vi "Command Editor Dialog.vi"(7 "Name (\"\" to Use Uuid)":string="Event CSM Tiny", 8 "Error In":errorcluster caption="Error in (no error)", 11 "CSM States":string="UI: Front Panel State >> Open -@ abc") -> (0 "Error Out":errorcluster, 3 "Command Out":string)   [LabVIEW 2017]
uses:
  _Support/Single-Line Type.ctl
  _Support/CSM Part Property.ctl
  _Support/Single-Line Selection Type.ctl
  <vilib>/Utility/miscctls.llb/LVRowAndColumnUnsignedTypeDef.ctl
  _Shared/Trim Single-line Text.vi
  AdvanceAPI/CSM - Break Down Multiple States String.vi
  AdvanceAPI/CSM - Compact Multiple States.vi
  AdvanceAPI/CSM - Keywords.vi
  _Polymophic/CSM - Filter Duplicated Lines.vi
  Communicable State Machine.lvlib
  _Shared/CSM Shared.lvlib
panel:
  out "MsgType":string
  out "Selction":string
  out "SelType":string
  out "Ref-String":string
  in  "clear arguments":bool
  in  "->|":bool
  in  "->":bool
  in  "-@":bool
  in  "Candidates":i32(listbox)
  # "Flood of Events:\n\nPanel/Pane Size Event\nSlide/Knob... User Event by dragging\nNumeric Control Value Change Event by Arraw Button"
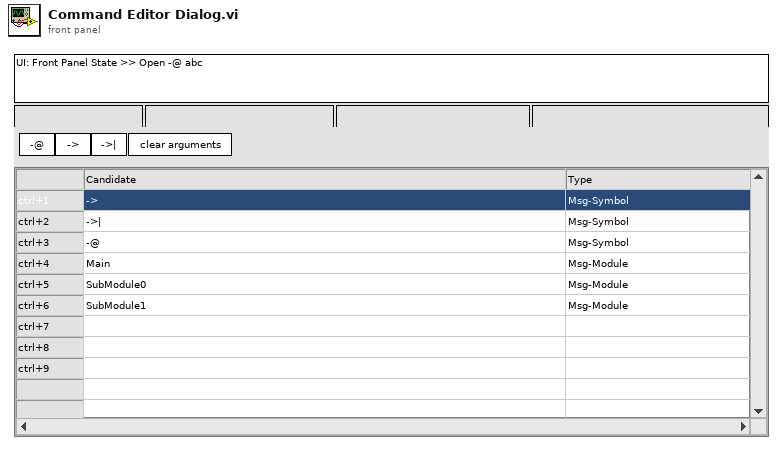
[diagram p1: front panel]
types:
  T1 = enum32{"Invalid", "Standard", "Closed", "Hidden", "Minimized", "Maximized"}
  T2 = enum32{"invalid app kind", "Development System", "Run Time System", "Student Edition", "Embedded LabVIEW", "Evaluation", "Custom"}
  T3 = typedef "LVRowAndColumnUnsignedTypeDef.ctl" = cluster{"Row":u32, "Column":u32}
  T4 = typedef "Communicable State Machine.lvlib/_CSM_Response Source Message.ctl" = cluster{"‘State":string, "’Arguments":string, "’Error":errorcluster}
  T5 = cluster{"Current VI Reference":refnum<vi>, "Close Panel on Exit?":bool}
  T6 = typedef "CSM Part Property.ctl" = cluster{"Section Start":u32, "Section End":u32, "Start":u32, "End":u32, "Section":string, "Core":string, "Sel Type":T7, "Ref-String":string}
  T7 = typedef "Single-Line Selection Type.ctl" = enum16{"<unknown>", "Reg-SourceSignal", "Reg-@Seperator", "Reg-ArgSymbol", "Reg-TargetAPI", "Reg-Module", "Reg-Symbol", "Reg-Oper", "Msg-State", "Msg-Arg", "Msg-ArgSymbol", "Msg-Symbol", "Msg-Module", "Broadcast-Signal", "Broadcast-ArgSymbol", "Broadcast-Arg", "Broadcast-Symbol", "Broadcast-Oper", "Comment-Symbol", "Comment-Content"}
  T8 = typedef "Single-Line Type.ctl" = enum16{"Message", "Broadcast", "Registration"}
  T9 = cluster{"Core":cluster{"Current VI Reference":refnum<vi>, "Close Panel on Exit?":bool}, "CSM States":string, "Selection":T6[], "Msg Type":T8}
  T10 = typedef "LVSelectionTypeDef.ctl" = cluster{"Selection Start":u32, "Selection End":u32}
  T11 = typedef "eventvkey.ctl" = enum16{"ASCII", "Enter", "Return", "Shift", "Ctrl", "Alt", "Cmd", "Opt", "Caps", "NumLock", "Clear", "Break", "Up", "Down", "Left", "Right", "Insert", "Delete", "Home", "End", "PageUp", "PageDown", "Escape", "Help", "Pause", "ScrollLock", "F1", "F2", "F3", "F4", "F5", "F6", "F7", "F8", "F9", "F10", "F11", "F12", "F13", "F14", "F15", "F16", "F17", "F18", "F19", "F20", "F21", "F22", "F23", "F24", "Play", "VolumeUp", "VolumeDown", "Mute", "Two Byte Char"}
  T12 = cluster{"Shift":bool, "Ctrl":bool, "Alt":bool, "Cmd":bool, "Opt":bool}
  T13 = typedef "LVPoint32TypeDef.ctl" = cluster{"Horizontal":i32, "Vertical":i32}
  T14 = typedef "LVRowAndColumnTypeDef.ctl" = cluster{"Row":i32, "Column":i32}
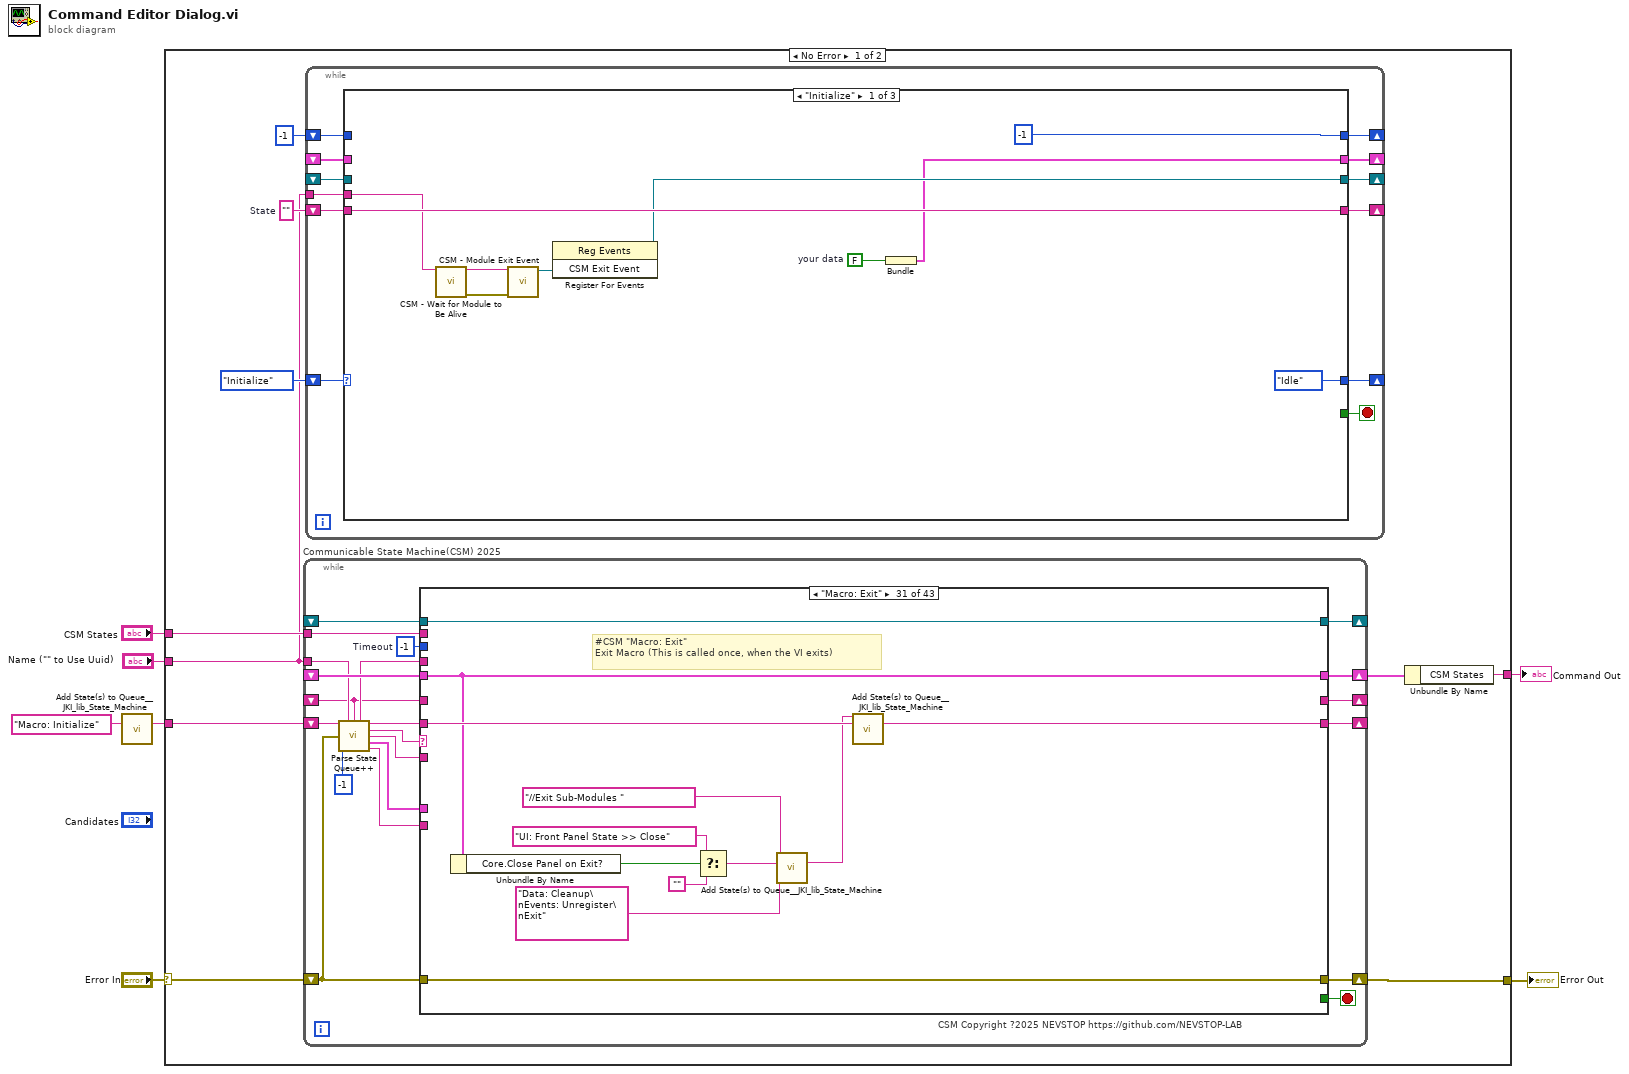
[diagram p0: block diagram]
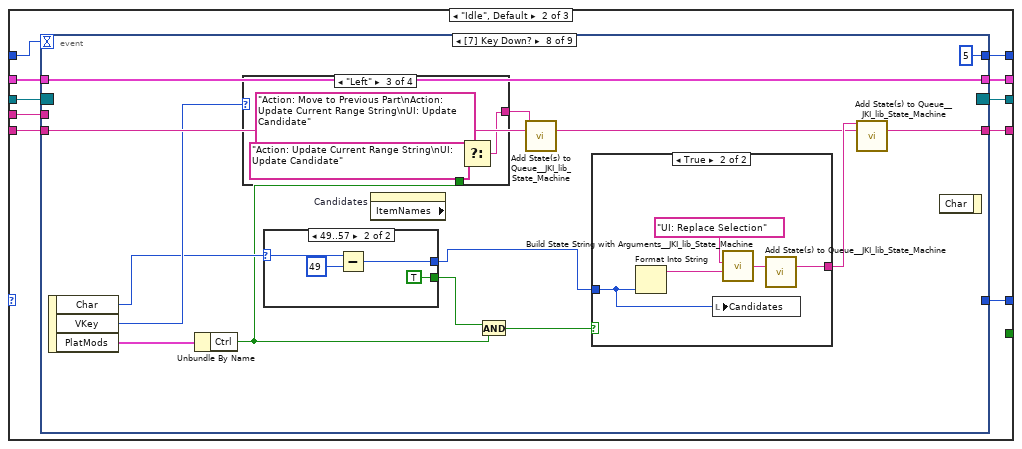
[diagram p2: hidden frame]
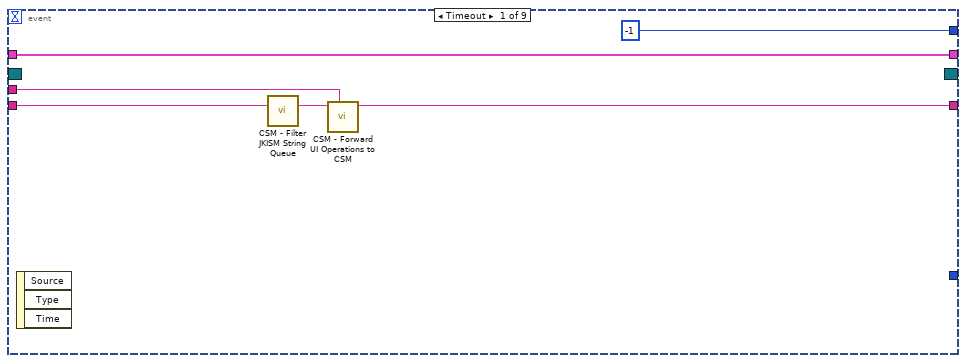
[diagram p3: hidden frame]
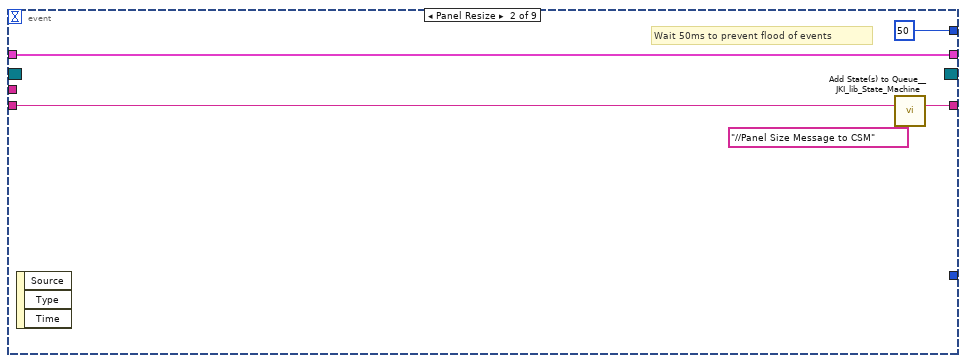
[diagram p4: hidden frame]
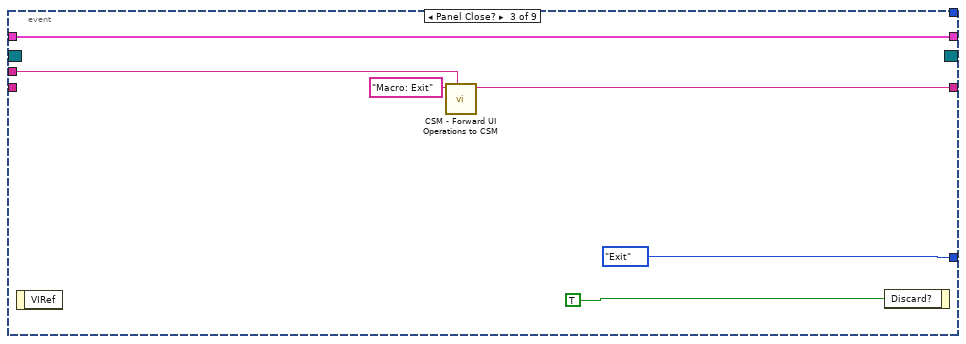
[diagram p5: hidden frame]
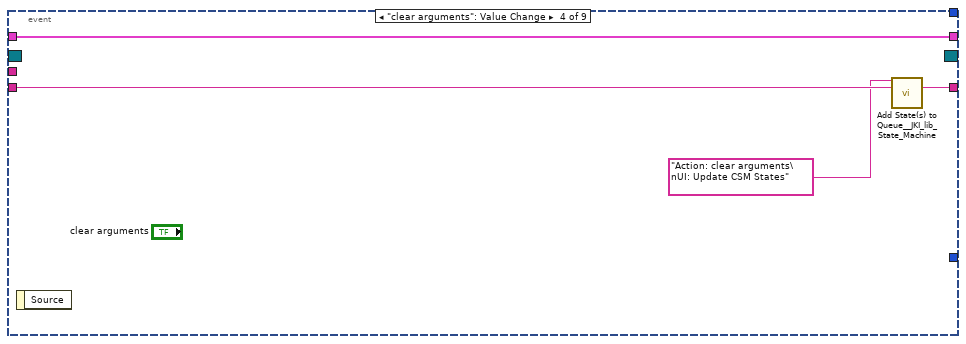
[diagram p6: hidden frame]
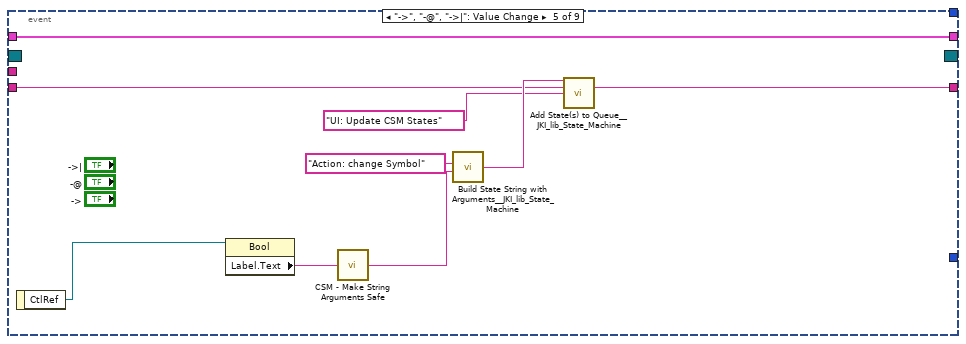
[diagram p7: hidden frame]
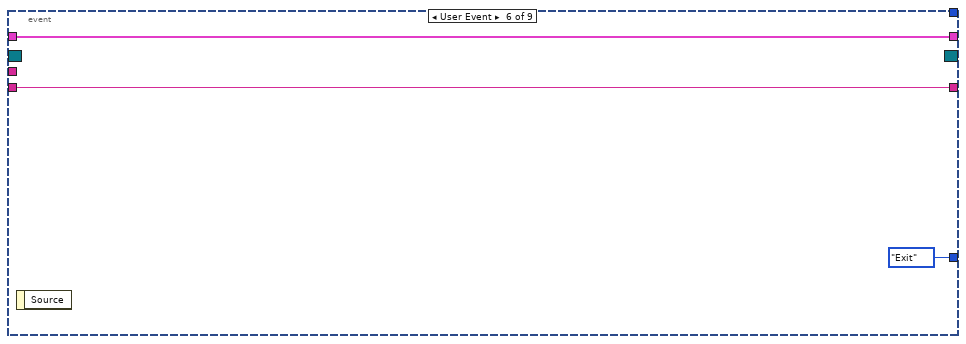
[diagram p8: hidden frame]
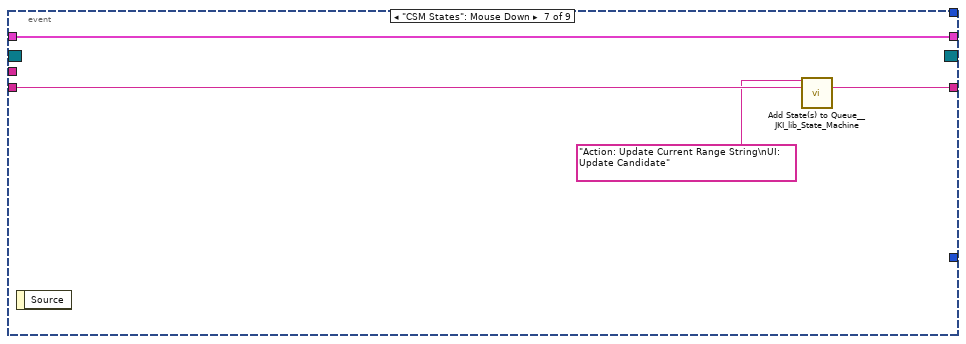
[diagram p9: hidden frame]
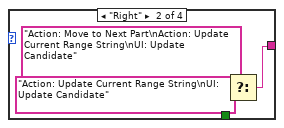
[diagram p11: hidden frame]
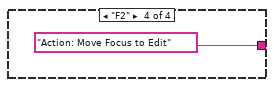
[diagram p12: hidden frame]
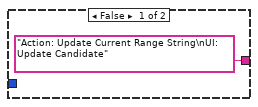
[diagram p13: hidden frame]
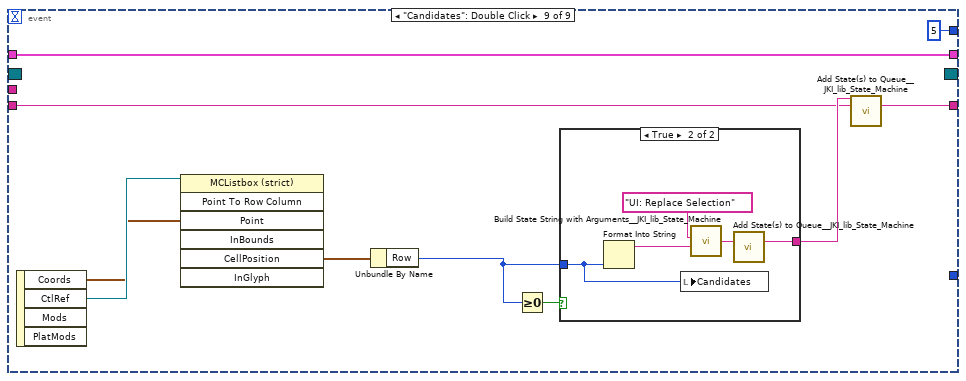
[diagram p15: hidden frame]
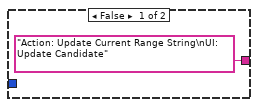
[diagram p16: hidden frame]
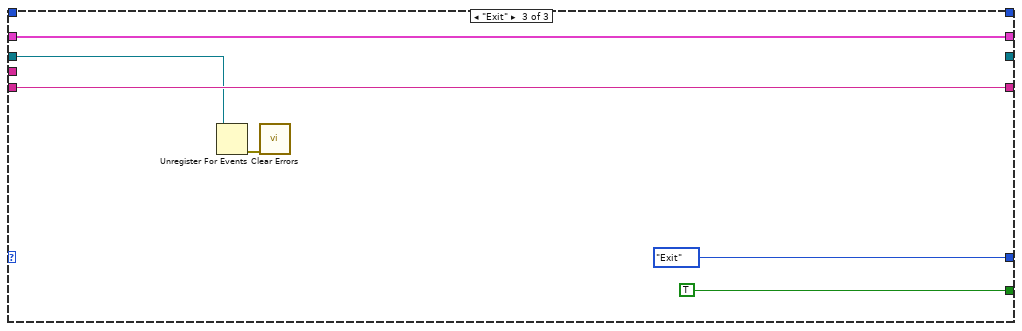
[diagram p17: hidden frame]
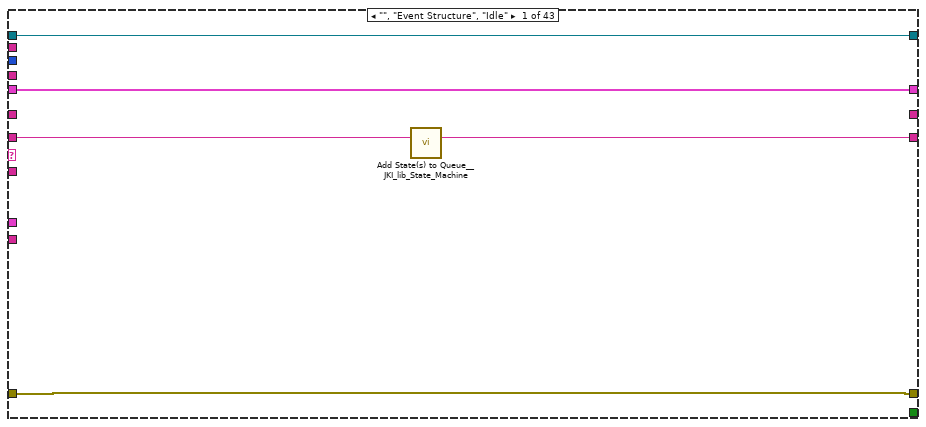
[diagram p18: hidden frame]
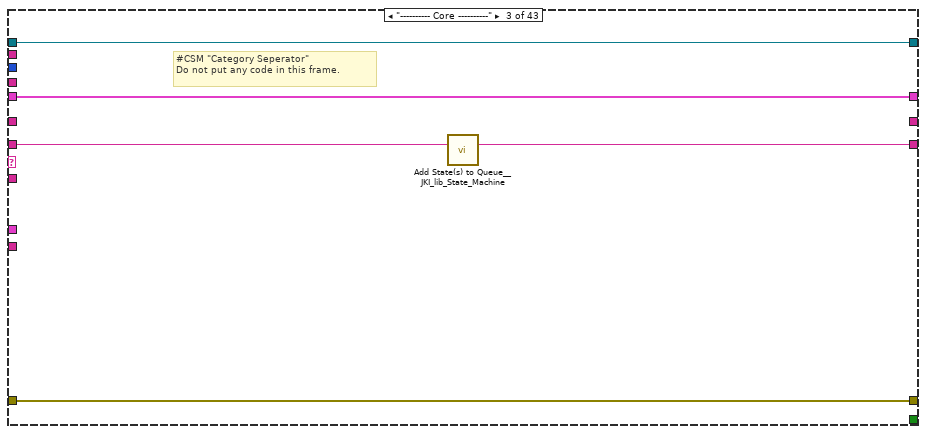
[diagram p20: hidden frame]
diagram:
  n1 = call <vilib>:"Add State(s) to Queue__JKI_lib_State_Machine.vi"("State(s) in (\"\")"="Macro: Initialize" ("Init State(\"Macro: Initialize\")")) -> ("States Out"=w7:string)  [unwired: 14 in]
  n2 = case shown="No Error" "Error In" {
    selector: "Error In" -> [w15 w682]
    tunnel: w7 -> [w17 _]
    tunnel: "Name (\"\" to Use Uuid)" -> [w8 _]
    tunnel: [w16 w682] -> w5
    tunnel: [w13 w681] -> w2
    tunnel: "CSM States" -> [w9 w681]
    frame No Error {
      w11 = ""  # State
      n3 = while "Communicable State Machine(CSM) 2025" {
        shift-right: [w157] -> w14
        shift-left: _ -> [w156]
        shift-right: [w160] -> w16
        shift-left: w15 -> [w154]
        shift-right: [w159] -> _
        shift-left: w17 -> [w161]
        tunnel: w8 -> [w150]
        shift-right: [w153] -> _
        shift-left: _ -> [w144]
        shift-right: [w152] -> _
        shift-left: _ -> [w151]
        tunnel: w9 -> [w143]
        stop <- w158 stop-if-true
        w155 = -1  # Timeout
        # "CSM Copyright ?2025 NEVSTOP https://github.com/NEVSTOP-LAB"
        n4 = call "Parse State Queue++.vi"("State Queue"=w161, "Name (\"\" to Use UUID)"=w150, "Response Arguments"=w144, "Previous Error"=w154, "Dequeue (1 ms)"=-1 ("Dequeue Timeout(0ms)")) -> ("Name Used"=w145:string, "Remaining States"=w162:string, "Current State"=w149:string, "Arguments"=w148:string, "Additional Information"=w147:T4, "Source CSM"=w146:string)  [unwired: 5 in]
        n5 = case shown="\"Macro: Exit\"" w149 {
          selector: w149 -> [_ _ _ w179 _ _ _ _ _ _ _ _ _ _ _ _ _ _ _ _ _ _ _ _ _ _ _ _ _ _ _ _ _ _ _ _ _ _ _ _ _ _ _]
          tunnel: w162 -> [w163 w170 w176 w184 w191 w197 w220 w226 w233 w242 w255 w270 w276 w281 w290 w297 w302 w309 w313 w319 w327 w338 w354 w427 w449 w453 w457 w468 w483 w489 w501 w504 w507 w519 w525 w534 w554 w582 w608 w625 w630 w639 w664]
          tunnel: w148 -> [_ _ _ _ _ w196 w215 w225 w232 w241 _ _ _ _ _ _ _ _ _ _ _ w333 w348 w425 _ _ _ _ _ _ _ _ w509 _ _ w526 w544 _ w602 _ _ _ _]
          tunnel: w156 -> [w165 w169 w173 w182 w190 w201 w221 w228 w235 w244 w254 w263 w274 w278 _ w292 w299 w308 w312 w316 w323 w336 w350 w435 w447 w452 w456 w464 w480 w486 w498 w503 w513 w518 w522 w532 w552 w580 w593 w619 w629 w638 w663]
          tunnel: [w166 w171 w174 w177 w192 errorcluster {"status"=FALSE, "code"=0, "source"=""} ("error out") w216 w223 w230 w247 w256 w267 w273 w279 w287 w293 w300 w303 w311 w317 w325 w334 w351 w436 w450 w454 w458 w469 w481 w487 w499 w505 w514 w520 w523 w535 w555 w583 w609 w626 w631 w640 w665] -> w160
          tunnel: w154 -> [w166 w171 w174 w185 w192 w198 w222 w224 w231 _ w256 w267 w273 w279 w287 w294 w300 _ w314 w317 w325 w335 w352 w436 w450 w454 w458 w469 w481 w487 w499 w505 w514 w520 w523 w535 w555 w583 w609 w626 w631 w640 w665]
          tunnel: [w167 w170 w175 w183 w191 w193 w219 w229 w236 w243 w255 w269 w275 w280 w289 w296 w301 w309 w313 w318 w326 w337 w353 w428 w449 w453 w457 w468 w482 w488 w500 w504 w508 w519 w524 w534 w554 w582 w608 w625 w630 w639 w664] -> w159
          tunnel: [_ _ _ _ _ _ TRUE _ _ _ _ _ TRUE _ _ _ _ _ _ _ _ _ _ _ _ _ _ _ _ _ _ _ _ _ _ _ _ _ _ _ _ _ _] -> w158
          tunnel: [w165 w169 w173 w182 w190 w201 w221 w228 w235 w245 w254 w268 w274 w278 w288 w292 w299 w308 w312 w316 w323 w336 w350 w435 w447 w452 w456 w464 w480 w486 w498 w503 w511 w518 w522 w529 w549 w577 w606 w618 w629 w638 w663] -> w157
          tunnel: w155 -> [_ _ _ _ _ _ _ _ _ _ _ _ _ _ _ _ _ _ _ _ _ _ _ _ _ _ _ _ _ _ _ _ _ _ _ _ _ _ _ _ _ _ _]
          tunnel: w146 -> [_ _ _ _ _ _ _ _ _ w239 _ _ _ _ _ _ _ _ _ _ _ _ _ _ _ _ _ _ _ _ _ _ _ _ _ _ _ _ _ _ _ _ _]
          tunnel: w147 -> [_ _ _ _ _ _ _ _ _ w246 _ _ _ _ _ _ _ _ _ _ _ _ _ _ _ _ _ _ _ _ _ _ _ _ _ _ _ _ _ _ _ _ _]
          tunnel: [_ _ _ "" w186 _ _ _ _ _ _ _ _ _ _ _ _ _ _ _ _ _ _ _ _ _ _ _ _ _ _ _ _ w515 _ _ _ _ _ _ _ _ _] -> w153
          tunnel: [w164 w168 w172 w180 w189 w200 w217 w227 w234 w248 w253 w257 w271 w277 w285 w291 w298 w307 w310 w315 w324 w332 w347 w434 w448 w451 w455 w467 w479 w484 w491 w502 w512 w517 w521 w533 w553 w581 w607 w624 w628 w637 w662] -> w152
          tunnel: w151 -> [w164 w168 w172 w180 w189 w200 w217 w227 w234 w248 w253 w257 w271 w277 w285 w291 w298 _ w310 w315 w324 w332 w347 w434 w448 w451 w455 w467 w479 w484 w491 w502 w512 w517 w521 w533 w553 w581 w607 w624 w628 w637 w662]
          tunnel: w145 -> [_ _ _ w178 _ _ w214 _ _ _ _ _ _ _ _ _ _ w306 _ _ _ _ _ _ _ _ _ _ _ _ _ _ _ _ _ _ _ _ _ _ _ _ _]
          tunnel: w144 -> [_ _ _ _ _ _ _ _ _ _ _ _ _ _ _ _ _ _ _ _ _ _ _ _ _ _ _ _ _ _ _ _ _ _ _ _ _ _ _ _ _ _ _]
          tunnel: w143 -> [_ _ _ _ _ _ _ _ _ _ _ _ _ _ w284 _ _ _ _ _ _ _ _ _ _ _ _ _ _ _ _ _ _ _ _ _ _ _ _ _ _ _ _]
          frame "", "Event Structure", "Idle" {
            n6 = call <vilib>:"Add State(s) to Queue__JKI_lib_State_Machine.vi"("State(s) in (\"\")"=w163) -> ("States Out"=w167:string)  [unwired: 14 in]
          }
          frame "CSM Documentation" {
          }
          frame "---------- Core ----------" {
            # "#CSM \"Category Seperator\"\nDo not put any code in this frame."
            n7 = call <vilib>:"Add State(s) to Queue__JKI_lib_State_Machine.vi"("State(s) in (\"\")"=w176) -> ("States Out"=w175:string)  [unwired: 14 in]
          }
          frame Default {
            # "#CSM \"Default\"\nthis is used to capture unhandled states and typos"
            # "Handle mistyped state name (developer tool)"
            n8 = call "CSM Unhandled State Error.vi"("error in (no error)"=w185, "Undefined State"=w179, "CSM Name"=w178) -> ("error out"=w177:errorcluster)  [unwired: 8 in]
            n9 = call <vilib>:"Add State(s) to Queue__JKI_lib_State_Machine.vi"("State(s) in (\"\")"=w184) -> ("States Out"=w183:string)  [unwired: 14 in]
          }
          frame "VI Reference" {
            n10 = Unbundle By Name(w190) -> ("Core"=w188:T5)
            n11 = Unbundle By Name(w188) -> ("Current VI Reference"=w187:refnum<vi>)
            n12 = call "CSM - Convert Data to HexStr.vi"("Variant"=w187) -> ("HEX String (0-9,A-F)"=w186:string)  [unwired: 8 in]
          }
          frame "Error Handler" {
            # "#CSM Disable this error dialog if you need"
            # "#CSM \"Error Handler\"\nYou can also output any states to clean-up after errors occur"
            # "Clear error"
            n13 = case shown="Error" w198 {
              selector: w198 -> [_ w208]
              tunnel: [w207 w210] -> w194
              tunnel: w197 -> [w207 w209]
              tunnel: w196 -> [w206 _]
              tunnel: [w205 w208] -> w199
              frame No Error {
                n14 = call "CSM - Convert Argument to Error.vi"("Argument"=w206) -> ("Error"=w205:errorcluster)  [unwired: 4 in]
                n15 = flat-sequence {
                  frame #0 {
                    # "#CSM External Error Handler Case\nUsually, it's because This CSM register others' \"Error Occurred\" status with \"Error Handler\". If other CSM have any error, the error will be passed here for central handling."
                  }
                }
              }
              frame Error {
                # "#CSM Internal Error Handler Case \nIf any error Occurred, \"Error Occurred\" \nstatus update will be broadcasted to system.\nParameter is Error Cluster."
                n16 = call "CSM - Convert Error to Argument.vi"("Error"=w208) -> ("Argument"=w212:string)  [unwired: 4 in]
                n17 = call <vilib>:"Build State String with Arguments__JKI_lib_State_Machine.vi"("Arguments (\"\")"=w212, "State"="Error Occurred" ("Status with Arguments")) -> ("State with Arguments"=w211:string)  [unwired: 4 in]
                n18 = call "CSM - Broadcast Status Change.vi"("Status With Arguments"=w211, "State Queue"=w209) -> ("Remaining States"=w210:string)  [unwired: 13 in]
              }
            }
            n19 = disable-structure shown="Enabled" {
              disable-tunnel: w199 -> [w203 w204]
              frame Enabled {
                n20 = call <vilib>:"General Error Handler.vi"("error in (no error)"=w203) -> ()  [unwired: 10 in, 5 out]
              }
              frame Disabled {
                n21 = call <vilib>:"Clear Errors.vi"("error in (no error)"=w204) -> ()  [unwired: 5 in, 2 out]
              }
            }
            n22 = call <vilib>:"Add State(s) to Queue__JKI_lib_State_Machine.vi"("State(s) in Front (\"\")"="// Post Error States", "State(s) in (\"\")"=w194) -> ("States Out"=w193:string)  [unwired: 13 in]
          }
          frame "Critical Error" {
            # "#CSM Stop in Critical Error\nWhen Critical Error occurs, Stop the loop immediately. Do NOT change this unless you fully understand the impact."
            # "#CSM \"Critical Error\"\nWhen any un-recoverable error occurs, CSM goes into this case."
            n23 = call "CSM Critical Error.vi"("error in (no error)"=w222, "Arugments (As Reason)"=w215, "CSM Name"=w214) -> ("error out"=w216:errorcluster)  [unwired: 8 in]
            n24 = call <vilib>:"Add State(s) to Queue__JKI_lib_State_Machine.vi"("State(s) in (\"\")"=w220) -> ("States Out"=w219:string)  [unwired: 14 in]
          }
          frame "Target Error" {
            # "#CSM \"Target Error\"\nWhen This CSM try to communicate with an un-existed CSM, This CSM goes into this case."
            n25 = call "CSM Target Error.vi"("error in (no error)"=w224, "Arguments (As CSM Name)"=w225) -> ("error out"=w223:errorcluster)  [unwired: 9 in]
            n26 = call <vilib>:"Add State(s) to Queue__JKI_lib_State_Machine.vi"("State(s) in (\"\")"=w226) -> ("States Out"=w229:string)  [unwired: 14 in]
          }
          frame "Target Timeout Error" {
            # "#CSM \"Target Timeout Error\"\nWhen This CSM could not get the sync-call response in time, This CSM goes into this case."
            n27 = call "CSM Target Timeout Error.vi"("error in (no error)"=w231, "Arguments (As CSM Name)"=w232) -> ("error out"=w230:errorcluster)  [unwired: 9 in]
            n28 = call <vilib>:"Add State(s) to Queue__JKI_lib_State_Machine.vi"("State(s) in (\"\")"=w233) -> ("States Out"=w236:string)  [unwired: 14 in]
          }
          frame "Async Response", "Response" {
            n29 = Unbundle(w246) -> ("‘State"=w240:string, "’Arguments"=w238:string, "’Error"=w237:errorcluster)
            n30 = case shown="Default" w240 {
              tunnel: [w252] -> w247
              tunnel: w237 -> [w252]
              tunnel: [w251] -> w245
              tunnel: w244 -> [w251]
              tunnel: [w249] -> w243
              tunnel: w242 -> [w250]
              tunnel: w241 -> [_]
              tunnel: w239 -> [_]
              tunnel: w238 -> [_]
              frame Default {
                # "#CSM Response Comments\nAfter Message is executed, CSM goes to this state for receive the response.\n    For Async Message(->), \"Async Response\" is used. This CSM will goes to \"Async Message Posted\" immediately and receive the \"Async Response\" after the callee finishes the message.\n    For Sync Message(@),  This CSM will wait until the message is done and immediately goes to \"Response\""
                # "#CSM \"Async Response\"\nHandle Async-call Response (\"Async Response\" for ->)"
                # "#CSM \"Response\"\nHandle Sync-call Response (\"Response\" for -@)"
                n31 = call <vilib>:"Add State(s) to Queue__JKI_lib_State_Machine.vi"("State(s) in (\"\")"=w250) -> ("States Out"=w249:string)  [unwired: 14 in]
              }
            }
          }
          frame "Async Message Posted" {
            # "#CSM \"Async Message Posted\"\nAfter Async Message is posted (-> or ->| ), CSM goes to this state for post-action.\nYou can use Argument - State to tell which Async Message is called."
          }
          frame "Initialize Core Data" {
            # "#CSM \"Initialize Core Data\"\nThis is used to determine panel behavior on exit"
            # "originally closed?"
            # "exe?"
            # "If panel starts closed or is an EXE, then close it when we exit"
            n32 = property class="VI"() -> ("FP.State"=w260:T1)  [unwired: 2 in, 2 out]
            n33 = property class="App"() -> ("App.Kind"=w266:T2)  [unwired: 2 in, 2 out]
            n34 = control-ref of="Current VI Reference"() -> (w261:refnum<vi>)
            n35 = Equal?(x=w260, y=T1."Closed" ("Front Panel Window:State")) -> (x = y?=w258:bool)
            n36 = Equal?(x=w266, y=T2."Run Time System" ("Application:Kind")) -> (x = y?=w264:bool)
            n37 = Or(x=w258, y=w264) -> (x .or. y?=w262:bool)
            n38 = Bundle By Name(cluster=w263, "Core.Current VI Reference"=w261, "Core.Close Panel on Exit?"=w262) -> (w268:T9)
            n39 = call <vilib>:"Add State(s) to Queue__JKI_lib_State_Machine.vi"("State(s) in (\"\")"=w270) -> ("States Out"=w269:string)  [unwired: 14 in]
          }
          frame "Exit" {
            # "#CSM \"Exit\"\nCase for exiting the loop. No errors that occur here will be handled."
            n40 = call <vilib>:"Add State(s) to Queue__JKI_lib_State_Machine.vi"("State(s) in (\"\")"=w276) -> ("States Out"=w275:string)  [unwired: 14 in]
          }
          frame "---------- Data ----------" {
            # "#CSM \"Category Seperator\"\nDo not put any code in this frame."
            n41 = call <vilib>:"Add State(s) to Queue__JKI_lib_State_Machine.vi"("State(s) in (\"\")"=w281) -> ("States Out"=w280:string)  [unwired: 14 in]
          }
          frame "Data: Initialize" {
            w282 = T6[] []  # Selection
            w283 = Single-Line_Type."Registration"  # Msg Type
            w286 = T5 {"Current VI Reference"=refnum, "Close Panel on Exit?"=FALSE}  # Core
            n42 = call <vilib>:"Add State(s) to Queue__JKI_lib_State_Machine.vi"("State(s) in (\"\")"=w290) -> ("States Out"=w289:string)  [unwired: 14 in]
            n43 = Bundle("Core"=w286, "CSM States"=w284, "Selection"=w282, "Msg Type"=w283) -> (w288:T9)  [unwired: 1 in]
          }
          frame "Data: Cleanup" {
            # "Cleanup any data and references, here.\n(this is called automatically, by the Macro: Exit)"
            n44 = Unbundle By Name(w292) -> ("Core.Current VI Reference"=w295:refnum<vi>)
            n45 = Close Reference(reference=w295, error in (no error)=w294) -> (error out=w293:errorcluster)
            n46 = call <vilib>:"Add State(s) to Queue__JKI_lib_State_Machine.vi"("State(s) in (\"\")"=w297) -> ("States Out"=w296:string)  [unwired: 14 in]
          }
          frame "---------- Events ----------" {
            # "#CSM \"Category Seperator\"\nDo not put any code in this frame."
            n47 = call <vilib>:"Add State(s) to Queue__JKI_lib_State_Machine.vi"("State(s) in (\"\")"=w302) -> ("States Out"=w301:string)  [unwired: 14 in]
          }
          frame "Events: Register" {
            # "#CSM \"Events: Register\"\nRegister user event. New Message Event is registered to break CSM waiting in event structure by default."
            # "#CSM Register New Message Event\nRegister message event to break Waiting in Event structure."
            n48 = call "CSM - Get New State Notifier Event.vi"("Name (\"\" to Use UUID)"=w306) -> ("error out"=w304:errorcluster, "New State Notifier Event"=w305:refnum<user-event>)  [unwired: 9 in]
            n49 = register-events(error in=w304, w305) -> (reference out=w307:refnum<event-registration>, error out=w303:errorcluster)  [unwired: 1 in]
          }
          frame "Events: Unregister" {
            # "#CSM \"Events: Unregister\"\nUnregister user event."
            n50 = Unregister For Events(event registration refnum=w310, error in=w314) -> (error out=w311:errorcluster)
          }
          frame "---------- UI ----------" {
            # "#CSM \"Category Seperator\"\nDo not put any code in this frame."
            n51 = call <vilib>:"Add State(s) to Queue__JKI_lib_State_Machine.vi"("State(s) in (\"\")"=w319) -> ("States Out"=w318:string)  [unwired: 14 in]
          }
          frame "UI: Initialize" {
            n52 = for {
              N: 9 -> [_]
              tunnel: [w329] -> w321 mode=indexing
              i -> [w331]
              n53 = Increment(x=w331) -> (x+1=w328:i32)
              n54 = Format Into String(format string="ctrl+%d", w328) -> (resulting string=w329:string)  [unwired: 2 in, 1 out]
            }
            n55 = property on="Candidates" class="MCListbox (strict)"("RowHdrs[]"=w321, "TopLeft"=T3 {"Row"=0, "Column"=0} ("Top Left Visible Cell")) -> ()  [unwired: 2 in, 2 out]
            n56 = call <vilib>:"Add State(s) to Queue__JKI_lib_State_Machine.vi"("State(s) in (\"\")"=w327) -> ("States Out"=w326:string)  [unwired: 14 in]
          }
          frame "UI: Cursor Set" {
            # "#CSM \"UI: Cursor Set\"\nSet and Unset Cursor Busy.\n(Usage: \"UI: Cursor Set >> Busy|Idle\")"
            # "Argument"
            n57 = disable-structure shown="Default" {
              disable-tunnel: w335 -> [w341 w346]
              disable-tunnel: [w340 w346] -> w334
              disable-tunnel: w333 -> [w339 _]
              frame condition #0 (active) {
                n58 = case shown="\"Idle\", Default" w339 {
                  tunnel: w341 -> [w343 w345]
                  tunnel: [w342 w344] -> w340
                  frame "Idle", Default {
                    n59 = call <vilib>:"Unset Busy.vi"("error in (no error)"=w343) -> ("error out"=w342:errorcluster)  [unwired: 10 in]
                  }
                  frame "Busy" {
                    n60 = call <vilib>:"Set Busy.vi"("error in (no error)"=w345) -> ("error out"=w344:errorcluster)  [unwired: 9 in, 1 out]
                  }
                }
              }
              frame condition #1 {
              }
            }
            n61 = call <vilib>:"Add State(s) to Queue__JKI_lib_State_Machine.vi"("State(s) in (\"\")"=w338) -> ("States Out"=w337:string)  [unwired: 14 in]
          }
          frame "UI: Front Panel State" {
            # "#CSM \"UI: Front Panel State\"\nSet Front Panel Open or Closed\n(Usage: \"UI: Front Panel State >> Open|Close\")"
            # "Argument"
            n62 = Unbundle By Name(w350) -> ("Core.Current VI Reference"=w349:refnum<vi>)
            n63 = call <vilib>:"Add State(s) to Queue__JKI_lib_State_Machine.vi"("State(s) in (\"\")"=w354) -> ("States Out"=w353:string)  [unwired: 14 in]
            n64 = case shown="\"Close\", \"Closed\"" w348 {
              tunnel: w352 -> [w360 w375 w386 w399 w412]
              tunnel: [w362 w376 w388 w401 w414] -> w351
              tunnel: w349 -> [w361 w373 w387 w400 w413]
              frame "Open", "Standard", Default {
                w355 = T1."Standard" ("State")
                n65 = property class="VI"(reference=w361, error in=w360) -> (reference out=w358:refnum<vi>, error out=w359:errorcluster, "FP.State"=w357:T1)
                n66 = Not Equal?(x=w357, y=w355) -> (x != y?=w356:bool)
                n67 = case shown="True" w356 {
                  tunnel: [w366 w368] -> w362
                  tunnel: w359 -> [w365 w368]
                  tunnel: w358 -> [w364 _]
                  tunnel: w355 -> [w363 _]
                  frame True {
                    n68 = invoke class="VI" method="FP.Open"(reference=w364, error in=w365, "Activate"=TRUE, "State"=w363) -> (error out=w366:errorcluster)  [unwired: 1 in, 4 out]
                  }
                  frame False {
                  }
                }
              }
              frame "Close", "Closed" {
                n69 = property class="VI"(reference=w373, error in=w375) -> (reference out=w372:refnum<vi>, error out=w374:errorcluster, "FP.State"=w370:T1)
                n70 = Not Equal?(x=w370, y=T1."Closed" ("Front Panel Window:State")) -> (x != y?=w369:bool)
                n71 = case shown="False" w369 {
                  tunnel: [w377 w380] -> w376
                  tunnel: w374 -> [w377 w379]
                  tunnel: w372 -> [_ w378]
                  frame False {
                  }
                  frame True {
                    n72 = invoke class="VI" method="FP.Close"(reference=w378, error in=w379) -> (error out=w380:errorcluster)  [unwired: 1 in, 2 out]
                  }
                }
              }
              frame "Hidden", "Hide" {
                w381 = T1."Hidden" ("State")
                n73 = property class="VI"(reference=w387, error in=w386) -> (reference out=w384:refnum<vi>, error out=w385:errorcluster, "FP.State"=w383:T1)
                n74 = Not Equal?(x=w383, y=w381) -> (x != y?=w382:bool)
                n75 = case shown="True" w382 {
                  tunnel: [w392 w393] -> w388
                  tunnel: w385 -> [w391 w393]
                  tunnel: w384 -> [w390 _]
                  tunnel: w381 -> [w389 _]
                  frame True {
                    n76 = invoke class="VI" method="FP.Open"(reference=w390, error in=w391, "State"=w389) -> (error out=w392:errorcluster)  [unwired: 2 in, 4 out]
                  }
                  frame False {
                  }
                }
              }
              frame "Minimize", "Minimized" {
                w394 = T1."Minimized" ("State")
                n77 = property class="VI"(reference=w400, error in=w399) -> (reference out=w397:refnum<vi>, error out=w398:errorcluster, "FP.State"=w396:T1)
                n78 = Not Equal?(x=w396, y=w394) -> (x != y?=w395:bool)
                n79 = case shown="True" w395 {
                  tunnel: [w405 w406] -> w401
                  tunnel: w398 -> [w404 w406]
                  tunnel: w397 -> [w403 _]
                  tunnel: w394 -> [w402 _]
                  frame True {
                    n80 = invoke class="VI" method="FP.Open"(reference=w403, error in=w404, "State"=w402) -> (error out=w405:errorcluster)  [unwired: 2 in, 4 out]
                  }
                  frame False {
                  }
                }
              }
              frame "Maximize", "Maximized" {
                w407 = T1."Maximized" ("State")
                n81 = property class="VI"(reference=w413, error in=w412) -> (reference out=w410:refnum<vi>, error out=w411:errorcluster, "FP.State"=w409:T1)
                n82 = Not Equal?(x=w409, y=w407) -> (x != y?=w408:bool)
                n83 = case shown="True" w408 {
                  tunnel: [w418 w419] -> w414
                  tunnel: w411 -> [w417 w419]
                  tunnel: w410 -> [w416 _]
                  tunnel: w407 -> [w415 _]
                  frame True {
                    n84 = invoke class="VI" method="FP.Open"(reference=w416, error in=w417, "State"=w415) -> (error out=w418:errorcluster)  [unwired: 2 in, 4 out]
                  }
                  frame False {
                  }
                }
              }
            }
          }
          frame "UI: Replace Selection" {
            n85 = Scan From String(input string=w425, default 1=-1 ("default value 1")) -> (output 1=w422:i32)  [unwired: 3 in, 3 out]
            n86 = Less Than 0?(x=w422) -> (x < 0?=w423:bool)
            n87 = property on="Candidates" class="MCListbox (strict)"() -> ("ItemNames"=w432:string[][], "Value"=w421:i32)  [unwired: 2 in, 2 out]
            n88 = Select(t=w421, s=w423, f=w422) -> (s? t:f=w420:i32)
            n89 = Index Array(array=w432, index (row)=w420, index (col)=0 ("disabled index (col)")) -> (element=w430:string)
            n90 = Empty String/Path?(string/path=w430) -> (empty?=w431:bool)
            n91 = Not(x=w431) -> (.not. x?=w433:bool)
            n92 = case shown="True" w433 {
              tunnel: w430 -> [_ w443]
              tunnel: ["Action: Update Current Range String\nUI: Update Candidate" ("States Out") w440] -> w426
              frame False {
              }
              frame True {
                n93 = call "CSM - Make String Arguments Safe.vi"("Argument String"=w443) -> ("Safe Argument String"=w439:string)  [unwired: 8 in]
                n94 = call <vilib>:"Build State String with Arguments__JKI_lib_State_Machine.vi"("Arguments (\"\")"=w439, "State"="Action: Replace Selction") -> ("State with Arguments"=w441:string)  [unwired: 4 in]
                n95 = call <vilib>:"Add State(s) to Queue__JKI_lib_State_Machine.vi"("State(s) in (\"\")"=w441, "State(s) at Back (\"\")"="Action: Update Current Range String" ("State(s) at Back (\"\")")) -> ("States Out"=w440:string)  [unwired: 13 in]
              }
            }
            n96 = call <vilib>:"Add State(s) to Queue__JKI_lib_State_Machine.vi"("State(s) in Front (\"\")"=w426, "State(s) in (\"\")"=w427) -> ("States Out"=w428:string)  [unwired: 13 in]
          }
          frame "UI: Update CSM States" {
            n97 = Unbundle By Name(w447) -> ("CSM States"=w445:string)
            n98 = control-ref of="CSM States"() -> (w446:refnum<vi>)
            n99 = property class="Str"(reference=w446, "Value"=w445) -> (reference out=w444:refnum<vi>)  [unwired: 1 in, 1 out]
            n100 = call "_Highlight CSM Scripts(StringControl).vi"("String Ctrl"=w444) -> ()  [unwired: 10 in, 1 out]
          }
          frame "UI: Update CSM Candidates" {
          }
          frame "UI: Update CSM-VI Candidates" {
          }
          frame "UI: Update Candidate" {
            n101 = Unbundle By Name(w464) -> ("Selection"=w463:T6[])
            n102 = for {
              tunnel: w463 -> [w478] mode=indexing
              tunnel: [w471] -> w459 mode=concatenating
              tunnel: [w470] -> w460 mode=concatenating
              n103 = Unbundle By Name(w478) -> ("Sel Type"=w477:T7)
              n104 = call "_scriptEditor.Input Candidates.vi"("Selection"=w478) -> ("Array"=w472:string[])  [unwired: 10 in]
              n105 = call "Remove Duplicates From StrArray.vi"("StrArray In"=w472) -> ("StrArray"=w470:string[])  [unwired: 9 in, 1 out]
              n106 = Format Into String(w477) -> (resulting string=w476:string)  [unwired: 3 in, 1 out]
              n107 = Array Size(array=w470) -> (size(s)=w475:i32)
              n108 = Initialize Array(w476, w475) -> (w474:string[])
              n109 = Build Array(w470, w474) -> (w473:string[][])
              n110 = Transpose 2D Array(2D array=w473) -> (transposed array=w471:string[][])
            }
            n111 = Index Array(array=w463) -> (element=w462:T6)  [unwired: 1 in]
            n112 = Unbundle By Name(w462) -> ("Section"=w461:string)
            n113 = call <vilib>:"Trim Whitespace.vi"("string"=w461) -> ("trimmed string"=w466:string)  [unwired: 1 in]
            n114 = Search 1D Array(1D array=w460, element=w466) -> (index of element=w465:i32)  [unwired: 1 in]
            n115 = property on="Candidates" class="MCListbox (strict)"("ItemNames"=w459, "Value"=w465) -> ()  [unwired: 2 in, 2 out]
          }
          frame "---------- Macro ----------" {
            # "#CSM \"Category Seperator\"\nDo not put any code in this frame."
            n116 = call <vilib>:"Add State(s) to Queue__JKI_lib_State_Machine.vi"("State(s) in (\"\")"=w483) -> ("States Out"=w482:string)  [unwired: 14 in]
          }
          frame "Macro: Initialize" {
            # "#CSM \"Macro: Initialize\"\nInitialization Macro (This is called once, when the VI starts)"
            n117 = call <vilib>:"Add State(s) to Queue__JKI_lib_State_Machine.vi"("State(s) in Front (\"\")"="Data: Initialize\nInitialize Core Data\nEvents: Register\nUI: Initialize\n//UI: Front Panel State >> Open\nUI: Update CSM States", "State(s) in (\"\")"=w489) -> ("States Out"=w488:string)  [unwired: 13 in]
          }
          frame "Macro: Exit" {
            # "#CSM \"Macro: Exit\"\nExit Macro (This is called once, when the VI exits)"
            n118 = Unbundle By Name(w498) -> ("Core.Close Panel on Exit?"=w497:bool)
            n119 = Select(t="UI: Front Panel State >> Close", s=w497, f="") -> (s? t:f=w494:string)
            n120 = call <vilib>:"Add State(s) to Queue__JKI_lib_State_Machine.vi"("State(s) in Front (\"\")"="//Exit Sub-Modules ", "State(s) in (\"\")"=w494, "State(s) at Back (\"\")"="Data: Cleanup\nEvents: Unregister\nExit") -> ("States Out"=w492:string)  [unwired: 12 in]
            n121 = call <vilib>:"Add State(s) to Queue__JKI_lib_State_Machine.vi"("State(s) in Front (\"\")"=w492, "State(s) in (\"\")"=w501) -> ("States Out"=w500:string)  [unwired: 13 in]
          }
          frame "---------- API ----------" {
            # "#CSM \"Category Seperator\"\nDo not put any code in this frame."
          }
          frame "API: Set Command" {
            # "#CSM API Example\nCopy/Rename this case for your own API"
            n122 = call "CSM - Revert Arguments-Safe String.vi"("Safe Argument String"=w509) -> ("Origin Argument String"=w510:string)  [unwired: 8 in]
            n123 = Bundle By Name(cluster=w513, "CSM States"=w510) -> (w511:T9)
            n124 = call <vilib>:"Add State(s) to Queue__JKI_lib_State_Machine.vi"("State(s) in (\"\")"=w507, "State(s) at Back (\"\")"="UI: Update CSM States" ("State(s) in Front (\"\")")) -> ("States Out"=w508:string)  [unwired: 13 in]
          }
          frame "API: Get Command" {
            n125 = local read "CSM States"() -> (w516:string)
            n126 = call "CSM - Make String Arguments Safe.vi"("Argument String"=w516) -> ("Safe Argument String"=w515:string)  [unwired: 8 in]
          }
          frame "---------- Action ----------" {
            # "#CSM \"Category Seperator\"\nDo not put any code in this frame."
            n127 = call <vilib>:"Add State(s) to Queue__JKI_lib_State_Machine.vi"("State(s) in (\"\")"=w525) -> ("States Out"=w524:string)  [unwired: 14 in]
          }
          frame "Action: Change Comments" {
            n128 = Unbundle By Name(w532) -> ("CSM States"=w531:string)
            n129 = Match Pattern(string=w531, regular expression="//") -> (before substring=w528:string)  [unwired: 1 in, 3 out]
            n130 = call "Concatenate State with Comments.vi"("Comments"=w526, "State"=w528) -> ("State With Arguments"=w527:string)  [unwired: 6 in]
            n131 = Bundle By Name(cluster=w532, "CSM States"=w527) -> (w529:T9)
          }
          frame "Action: change Symbol" {
            w539 = " " ("regular expression")
            n132 = Unbundle By Name(w552) -> ("CSM States"=w551:string)
            n133 = Match Pattern(string=w551, regular expression="//") -> (before substring=w547:string, after substring=w548:string)  [unwired: 1 in, 2 out]
            n134 = for {
              tunnel: w547 -> [w562]
              tunnel: string[] ["->|", "-@", "->"] ("regular expression") -> [w561] mode=indexing
              tunnel: [w559] -> _ if=w558
              tunnel: [w557] -> w545
              tunnel: [w556] -> w540
              stop <- w558 stop-if-true
              n135 = Match Pattern(string=w562, regular expression=w561) -> (before substring=w557:string, match substring=w559:string, after substring=w556:string, offset past match=w560:i32)  [unwired: 1 in]
              n136 = Greater Or Equal To 0?(x=w560) -> (x >= 0?=w558:bool)
            }
            n137 = call "CSM - Revert Arguments-Safe String.vi"("Safe Argument String"=w544) -> ("Origin Argument String"=w543:string)  [unwired: 8 in]
            n138 = call <vilib>:"Trim Whitespace.vi"("string"=w545) -> ("trimmed string"=w542:string)  [unwired: 1 in]
            n139 = call <vilib>:"Trim Whitespace.vi"("string"=w540) -> ("trimmed string"=w541:string)  [unwired: 1 in]
            n140 = call <vilib>:"Trim Whitespace.vi"("string"=w548) -> ("trimmed string"=w536:string)  [unwired: 1 in]
            n141 = Concatenate Strings(w542, w539, w543, w539, w541) -> (w537:string)
            n142 = call "Concatenate State with Comments.vi"("Comments"=w536, "State"=w537) -> ("State With Arguments"=w538:string)  [unwired: 6 in]
            n143 = Bundle By Name(cluster=w552, "CSM States"=w538) -> (w549:T9)
          }
          frame "Action: clear arguments" {
            w573 = " " ("regular expression")
            n144 = Unbundle By Name(w580) -> ("CSM States"=w579:string)
            n145 = Match Pattern(string=w579, regular expression="//") -> (before substring=w575:string, after substring=w576:string)  [unwired: 1 in, 2 out]
            n146 = for {
              tunnel: w575 -> [w590]
              tunnel: string[] ["->|", "-@", "->"] ("regular expression") -> [w589] mode=indexing
              tunnel: [w587] -> w569 if=w586
              tunnel: [w585] -> w571
              tunnel: [w584] -> w564
              stop <- w586 stop-if-true
              n147 = Match Pattern(string=w590, regular expression=w589) -> (before substring=w585:string, match substring=w587:string, after substring=w584:string, offset past match=w588:i32)  [unwired: 1 in]
              n148 = Greater Or Equal To 0?(x=w588) -> (x >= 0?=w586:bool)
            }
            n149 = call <vilib>:"Trim Whitespace.vi"("string"=w576) -> ("trimmed string"=w566:string)  [unwired: 1 in]
            n150 = Match Pattern(string=w571, regular expression=">>") -> (before substring=w565:string)  [unwired: 1 in, 3 out]
            n151 = call <vilib>:"Trim Whitespace.vi"("string"=w564) -> ("trimmed string"=w563:string)  [unwired: 1 in]
            n152 = call <vilib>:"Build State String with Arguments__JKI_lib_State_Machine.vi"("State"=w565) -> ("State with Arguments"=w570:string)  [unwired: 5 in]
            n153 = Concatenate Strings(w570, w573, w569, w573, w563) -> (w567:string)
            n154 = call "Concatenate State with Comments.vi"("Comments"=w566, "State"=w567) -> ("State With Arguments"=w568:string)  [unwired: 6 in]
            n155 = Bundle By Name(cluster=w580, "CSM States"=w568) -> (w577:T9)
          }
          frame "Action: Replace Selction" {
            n156 = Unbundle By Name(w593) -> ("Selection"=w592:T6[])
            n157 = Index Array(array=w592) -> (element=w591:T6)  [unwired: 1 in]
            n158 = property on="CSM States" class="Str"() -> ("Value"=w601:string)  [unwired: 2 in, 2 out]
            n159 = Unbundle By Name(w591) -> ("Start"=w604:u32, "End"=w605:u32)
            n160 = call "CSM - Revert Arguments-Safe String.vi"("Safe Argument String"=w602) -> ("Origin Argument String"=w598:string)  [unwired: 8 in]
            n161 = Subtract(x=w605, y=w604) -> (x-y=w603:u32)
            n162 = control-ref of="CSM States"() -> (w599:refnum<vi>)
            n163 = Replace Substring(2:w603, 3:w604, 4:w598, 5:w601) -> (1:w597:string)  [unwired: 1 out]
            n164 = property class="Str"(reference=w599, "Value"=w597) -> (reference out=w596:refnum<vi>)  [unwired: 1 in, 1 out]
            n165 = Search/Split String(string=w597, search string/char (-)=w598) -> (offset of match=w594:i32)  [unwired: 1 in, 2 out]
            n166 = String Length(string=w598) -> (length=w600:i32)
            n167 = call "_Highlight CSM Scripts(StringControl).vi"("String Ctrl"=w596) -> ()  [unwired: 10 in, 1 out]
            n168 = Add(x=w594, y=w600) -> (x+y=w595:i32)
            n169 = Bundle By Name(cluster=w593, "Msg Type"=w595, "CSM States"=w597) -> (w606:T9)
          }
          frame "Action: Update Current Range String" {
            n170 = control-ref of="CSM States"() -> (w622:refnum<vi>)
            n171 = property class="Str"(reference=w622) -> ("Value"=w623:string, "Text.Selection"=w621:T10)  [unwired: 1 in, 2 out]
            n172 = Unbundle By Name(w621) -> ("Selection Start"=w620:u32)
            n173 = call "CSM Part Property at Cursor.vi"("Pos"=w620, "Single-line Text"=w623) -> ("Msg Type"=w617:T8, "Property"=w610:T6[])  [unwired: 7 in, 1 out]
            n174 = Index Array(array=w610) -> (element=w614:T6)  [unwired: 1 in]
            n175 = Unbundle By Name(w614) -> ("Section"=→"Selction":string, "Sel Type"=w612:T7, "Ref-String"=→"Ref-String":string)
            n176 = Bundle By Name(cluster=w619, "Selection"=w610, "Msg Type"=w617) -> (w618:T9)
            n177 = Format Into String(w617) -> (resulting string=→"MsgType":string)  [unwired: 3 in, 1 out]
            n178 = Format Into String(w612) -> (resulting string=→"SelType":string)  [unwired: 3 in, 1 out]
          }
          frame "Action: Move Focus to Edit" {
            n179 = property on="CSM States" class="Str"("Key Focus"=TRUE) -> ()  [unwired: 2 in, 2 out]
          }
          frame "Action: Move to Next Part" {
            n180 = property on="CSM States" class="Str"() -> ("Value"=w633:string, "Key Focus"=w636:bool, "Text.Selection End"=w635:u32, "Text.Selection Start"=w634:u32)  [unwired: 2 in, 2 out]
            n181 = Max & Min(x=w635, y=w634) -> (min(x,y)=w632:u32)  [unwired: 1 out]
            n182 = case shown="True" w636 {
              tunnel: w633 -> [_ w648]
              tunnel: w632 -> [_ w647]
              frame False {
              }
              frame True {
                n183 = call "Single-Line To CSM Parts.vi"("Single-line Text"=w648) -> ("Property"=w646:T6[])  [unwired: 7 in, 3 out]
                n184 = for {
                  tunnel: w647 -> [w656]
                  tunnel: w646 -> [w651] mode=indexing
                  tunnel: [w651] -> _ mode=indexing if=w649
                  tunnel: [w650] -> w645 mode=indexing if=w649
                  i -> [w650]
                  n185 = Unbundle By Name(w651) -> ("Section Start"=w652:u32, "Section End"=w653:u32)
                  n186 = Greater Or Equal?(x=w656, y=w652) -> (x >= y?=w654:bool)
                  n187 = Less Or Equal?(x=w656, y=w653) -> (x <= y?=w655:bool)
                  n188 = And(x=w655, y=w654) -> (x .and. y?=w649:bool)
                }
                n189 = Array Max & Min(array=w645) -> (max value=w644:i32)  [unwired: 3 out]
                n190 = Increment(x=w644) -> (x+1=w643:i32)
                n191 = Index Array(array=w646, index=w643) -> (element=w642:T6)
                n192 = Unbundle By Name(w642) -> ("Start"=w641:u32)
                n193 = property on="CSM States" class="Str"("Text.Selection End"=w641, "Text.Selection Start"=w641) -> ()  [unwired: 2 in, 2 out]
              }
            }
          }
          frame "Action: Move to Previous Part" {
            n194 = property on="CSM States" class="Str"() -> ("Value"=w658:string, "Key Focus"=w661:bool, "Text.Selection End"=w660:u32, "Text.Selection Start"=w659:u32)  [unwired: 2 in, 2 out]
            n195 = Max & Min(x=w660, y=w659) -> (min(x,y)=w657:u32)  [unwired: 1 out]
            n196 = case shown="True" w661 {
              tunnel: w658 -> [_ w672]
              tunnel: w657 -> [_ w671]
              frame False {
              }
              frame True {
                n197 = call "Single-Line To CSM Parts.vi"("Single-line Text"=w672) -> ("Property"=w670:T6[])  [unwired: 7 in, 3 out]
                n198 = for {
                  tunnel: w671 -> [w680]
                  tunnel: w670 -> [w675] mode=indexing
                  tunnel: [w675] -> _ mode=indexing if=w673
                  tunnel: [w674] -> w667 mode=indexing if=w673
                  i -> [w674]
                  n199 = Unbundle By Name(w675) -> ("Section Start"=w676:u32, "Section End"=w677:u32)
                  n200 = Greater Or Equal?(x=w680, y=w676) -> (x >= y?=w678:bool)
                  n201 = Less Or Equal?(x=w680, y=w677) -> (x <= y?=w679:bool)
                  n202 = And(x=w679, y=w678) -> (x .and. y?=w673:bool)
                }
                n203 = Array Max & Min(array=w667) -> (min value=w666:i32)  [unwired: 3 out]
                n204 = Index Array(array=w670, index=w666) -> (element=w669:T6)
                n205 = Unbundle By Name(w669) -> ("Start"=w668:u32)
                n206 = property on="CSM States" class="Str"("Text.Selection End"=w668, "Text.Selection Start"=w668) -> ()  [unwired: 2 in, 2 out]
              }
            }
          }
        }
      }
      n207 = while {
        shift-right: [w28] -> _
        shift-left: enum16{"Idle", "Initialize", "Exit"}."Initialize" -> [w29]
        tunnel: w8 -> [w26]
        shift-right: [w24] -> _
        shift-left: w11 -> [w25]
        shift-right: [w22] -> _
        shift-left: -1 -> [w23]
        shift-right: [w21] -> _
        shift-left: _ -> [w20]
        shift-right: [w19] -> _
        shift-left: _ -> [w18]
        stop <- w27 stop-if-true
        n208 = case shown="\"Initialize\"" w29 {
          tunnel: [enum16{"Idle", "Initialize", "Exit"}."Idle" w49 enum16{"Idle", "Initialize", "Exit"}."Exit"] -> w28
          tunnel: [_ _ TRUE] -> w27
          tunnel: w26 -> [w35 w48 _]
          tunnel: w25 -> [w38 w46 w139]
          tunnel: [w38 w47 w139] -> w24
          tunnel: w23 -> [_ w44 _]
          tunnel: [-1 w45 _] -> w22
          tunnel: [w34 w42 _] -> w21
          tunnel: w20 -> [_ w43 w138]
          tunnel: [w30 w40 w136] -> w19
          tunnel: w18 -> [_ w41 w136]
          frame "Initialize" {
            w31 = FALSE  # your data
            n209 = call "CSM - Wait for Module to Be Alive.vi"("CSM Name"=w35) -> ("CSM Name (Dup)"=w33:string, "error out"=w32:errorcluster)  [unwired: 12 in, 1 out]
            n210 = call "CSM - Module Exit Event.vi"("Error In"=w32, "Name (\"\" to Use UUID) In"=w33) -> ("CSM Exit Event"=w36:refnum<user-event>)  [unwired: 7 in, 2 out]
            n211 = register-events(w36) -> (reference out=w34:refnum<event-registration>)  [unwired: 2 in, 1 out]
            n212 = Bundle("your data"=w31) -> (w30:cluster{"your data":bool})  [unwired: 1 in]
          }
          frame "Idle", Default {
            n213 = event shown="[7] Key Down?" {
              selector: w43 -> [_ _ _ _ _ _ _ _ _]
              dyn-events: [_ _ _ _ _ _ _ _ _] -> w42
              timeout: w44 -> [_ _ _ _ _ _ _ _ _]
              tunnel: [_ _ enum16{"Idle", "Initialize", "Exit"}."Exit" _ _ enum16{"Idle", "Initialize", "Exit"}."Exit" _ _ _] -> w49
              tunnel: w48 -> [w53 _ w63 _ _ _ _ _ _]
              tunnel: w46 -> [w51 w60 _ w68 w73 w82 w84 w95 w125]
              tunnel: [w54 w59 w62 w69 w72 w82 w85 w94 w127] -> w47
              tunnel: [-1 50 _ _ _ _ _ 5 5] -> w45
              tunnel: w41 -> [w52 w56 w61 w70 w79 w80 w86 w100 w129]
              tunnel: [w52 w56 w61 w70 w79 w80 w86 w100 w129] -> w40
              event Timeout {
                n214 = event-data() -> ()  [unwired: 1 in, 3 out]
                n215 = call-poly "CSM - Filter JKISM String Queue.vi"("States In"=w51) -> ("States Out"=w50:string)  [unwired: 14 in]
                n216 = call "CSM - Forward UI Operations to CSM.vi"("Name (\"\" to Use UUID)"=w53, "State(s) In (\"\")"=w50) -> ("States Out"=w54:string)  [unwired: 8 in, 1 out]
              }
              event Panel Resize {
                # "Wait 50ms to prevent flood of events"
                n217 = event-data() -> ()  [unwired: 1 in, 3 out]
                n218 = call <vilib>:"Add State(s) to Queue__JKI_lib_State_Machine.vi"("State(s) in (\"\")"=w60, "State(s) at Back (\"\")"="//Panel Size Message to CSM" ("State(s) at Back (\"\")")) -> ("States Out"=w59:string)  [unwired: 13 in]
              }
              event Panel Close? {
                n219 = event-data() -> ()  [unwired: 1 in, 1 out]
                n220 = call "CSM - Forward UI Operations to CSM.vi"("Name (\"\" to Use UUID)"=w63, "State(s) In (\"\")"="Macro: Exit" ("State")) -> ("States Out"=w62:string)  [unwired: 8 in, 1 out]
                n221 = event-data("Discard?"=TRUE) -> ()  [unwired: 1 in, 1 out]
              }
              event "clear arguments": Value Change {
                n222 = event-data() -> ()  [unwired: 1 in, 1 out]
                n223 = call <vilib>:"Add State(s) to Queue__JKI_lib_State_Machine.vi"("State(s) in Front (\"\")"="Action: clear arguments\nUI: Update CSM States" ("State(s) in Front (\"\")"), "State(s) in (\"\")"=w68) -> ("States Out"=w69:string)  [unwired: 13 in]
              }
              event "->", "-@", "->|": Value Change {
                n224 = event-data() -> ("CtlRef"=w71:refnum<vi>)  [unwired: 1 in]
                n225 = property class="Bool"(reference=w71) -> ("Label.Text"=w76:string)  [unwired: 1 in, 2 out]
                n226 = call "CSM - Make String Arguments Safe.vi"("Argument String"=w76) -> ("Safe Argument String"=w75:string)  [unwired: 8 in]
                n227 = call <vilib>:"Build State String with Arguments__JKI_lib_State_Machine.vi"("Arguments (\"\")"=w75, "State"="Action: change Symbol") -> ("State with Arguments"=w78:string)  [unwired: 4 in]
                n228 = call <vilib>:"Add State(s) to Queue__JKI_lib_State_Machine.vi"("State(s) in Front (\"\")"=w78, "State(s) in (\"\")"=w73, "State(s) at Back (\"\")"="UI: Update CSM States" ("State")) -> ("States Out"=w72:string)  [unwired: 12 in]
              }
              event User Event {
                n229 = event-data() -> ()  [unwired: 1 in, 1 out]
              }
              event "CSM States": Mouse Down {
                n230 = event-data() -> ()  [unwired: 1 in, 1 out]
                n231 = call <vilib>:"Add State(s) to Queue__JKI_lib_State_Machine.vi"("State(s) in Front (\"\")"="Action: Update Current Range String\nUI: Update Candidate" ("State(s) at Back (\"\")"), "State(s) in (\"\")"=w84) -> ("States Out"=w85:string)  [unwired: 13 in]
              }
              event Key Down? {
                n232 = event-data() -> ("Char"=w91:i16, "VKey"=w92:T11, "PlatMods"=w93:T12)  [unwired: 1 in]
                n233 = Unbundle By Name(w93) -> ("Ctrl"=w90:bool)
                n234 = case shown="\"Left\"" w92 {
                  tunnel: [_ w102 w106 "Action: Move Focus to Edit" ("State(s) in Front (\"\")")] -> w96
                  tunnel: w90 -> [_ w101 w105 _]
                  frame "ASCII", Default {
                  }
                  frame "Right" {
                    n235 = Select(t="Action: Move to Next Part\nAction: Update Current Range String\nUI: Update Candidate" ("State(s) in Front (\"\")"), s=w101, f="Action: Update Current Range String\nUI: Update Candidate" ("State(s) in Front (\"\")")) -> (s? t:f=w102:string)
                  }
                  frame "Left" {
                    n236 = Select(t="Action: Move to Previous Part\nAction: Update Current Range String\nUI: Update Candidate" ("State(s) in Front (\"\")"), s=w105, f="Action: Update Current Range String\nUI: Update Candidate" ("State(s) in Front (\"\")")) -> (s? t:f=w106:string)
                  }
                  frame "F2" {
                  }
                }
                n237 = case shown="49..57" w91 {
                  selector: w91 -> [_ w119]
                  tunnel: [_ w117] -> w88
                  tunnel: [_ TRUE] -> w99
                  frame 0, Default {
                  }
                  frame 49..57 {
                    n238 = Subtract(x=w119, y=i16 49) -> (x-y=w117:i16)
                  }
                }
                n239 = property on="Candidates" class="MCListbox (strict)" props=["ItemNames"]() -> ()  [unwired: 2 in, 3 out]
                n240 = And(x=w99, y=w90) -> (x .and. y?=w87:bool)
                n241 = call <vilib>:"Add State(s) to Queue__JKI_lib_State_Machine.vi"("State(s) in Front (\"\")"=w96, "State(s) in (\"\")"=w95) -> ("States Out"=w97:string)  [unwired: 13 in]
                n242 = case shown="True" w87 {
                  tunnel: ["Action: Update Current Range String\nUI: Update Candidate" ("States Out") w113] -> w98
                  tunnel: w88 -> [_ w112]
                  frame False {
                  }
                  frame True {
                    n243 = Format Into String(w112) -> (resulting string=w111:string)  [unwired: 3 in, 1 out]
                    n244 = local write "Candidates"(w112) -> ()
                    n245 = call <vilib>:"Build State String with Arguments__JKI_lib_State_Machine.vi"("Arguments (\"\")"=w111, "State"="UI: Replace Selection") -> ("State with Arguments"=w114:string)  [unwired: 4 in]
                    n246 = call <vilib>:"Add State(s) to Queue__JKI_lib_State_Machine.vi"("State(s) in (\"\")"=w114) -> ("States Out"=w113:string)  [unwired: 14 in]
                  }
                }
                n247 = call <vilib>:"Add State(s) to Queue__JKI_lib_State_Machine.vi"("State(s) in Front (\"\")"=w98, "State(s) in (\"\")"=w97) -> ("States Out"=w94:string)  [unwired: 13 in]
                n248 = event-data() -> ()  [unwired: 2 in, 1 out]
              }
              event "Candidates": Double Click {
                n249 = event-data() -> ("Coords"=w122:T13, "CtlRef"=w124:refnum<vi>)  [unwired: 1 in, 2 out]
                n250 = invoke class="MCListbox (strict)" method="Point To Row Column"(reference=w124, "Point"=w122) -> ("CellPosition"=w121:T14)  [unwired: 5 in, 6 out]
                n251 = Unbundle By Name(w121) -> ("Row"=w120:i32)
                n252 = Greater Or Equal To 0?(x=w120) -> (x >= 0?=w123:bool)
                n253 = case shown="True" w123 {
                  tunnel: ["Action: Update Current Range String\nUI: Update Candidate" ("States Out") w133] -> w128
                  tunnel: w120 -> [_ w132]
                  frame False {
                  }
                  frame True {
                    n254 = Format Into String(w132) -> (resulting string=w131:string)  [unwired: 3 in, 1 out]
                    n255 = local write "Candidates"(w132) -> ()
                    n256 = call <vilib>:"Build State String with Arguments__JKI_lib_State_Machine.vi"("Arguments (\"\")"=w131, "State"="UI: Replace Selection") -> ("State with Arguments"=w134:string)  [unwired: 4 in]
                    n257 = call <vilib>:"Add State(s) to Queue__JKI_lib_State_Machine.vi"("State(s) in (\"\")"=w134) -> ("States Out"=w133:string)  [unwired: 14 in]
                  }
                }
                n258 = call <vilib>:"Add State(s) to Queue__JKI_lib_State_Machine.vi"("State(s) in Front (\"\")"=w128, "State(s) in (\"\")"=w125) -> ("States Out"=w127:string)  [unwired: 13 in]
              }
            }
          }
          frame "Exit" {
            n259 = Unregister For Events(event registration refnum=w138) -> (error out=w137:errorcluster)  [unwired: 1 in]
            n260 = call <vilib>:"Clear Errors.vi"("error in (no error)"=w137) -> ()  [unwired: 5 in, 2 out]
          }
        }
      }
      n261 = Unbundle By Name(w14) -> ("CSM States"=w13:string)
    }
    frame Error {
    }
  }
  "Error Out" <- w5
  "Command Out" <- w2
